vi "命令.vi"(10 "应用名称":string, 11 "选项":enum16{"归零", "自动", "退出", "关机"}(ring)) -> (3 "完成":bool)   [LabVIEW 2017]
panel:
  out "standard output 2":string caption="标准输出"
  out "匹配后偏移量 2":i32
  # "Google Chrome"
  # "SQLiteSpy.exe"
  # "Macromedia Flash Player 7.0  r14"
  # "動物連連看1.exe"
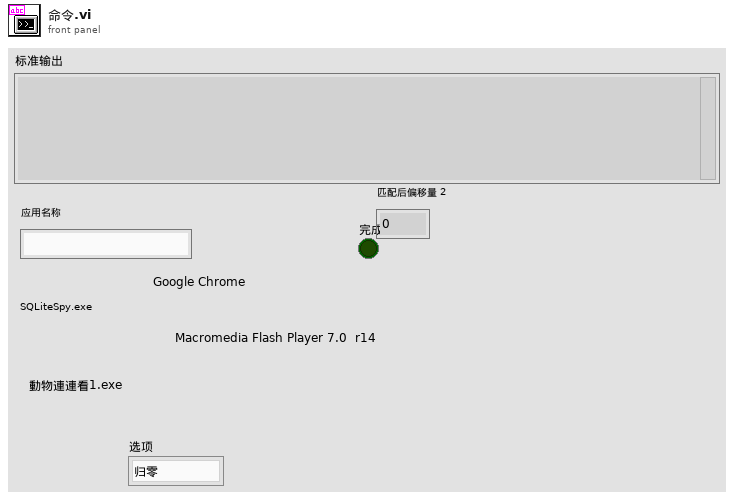
[diagram p1: front panel]
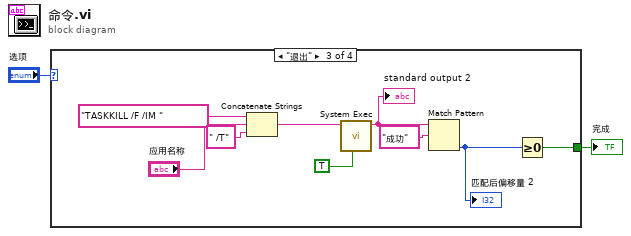
[diagram p0: block diagram]
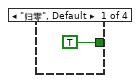
[diagram p2: hidden frame]
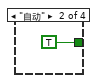
[diagram p3: hidden frame]
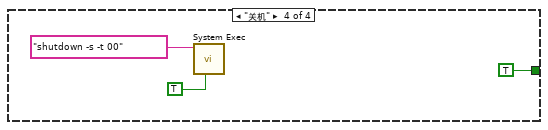
[diagram p4: hidden frame]
diagram:
  n1 = case shown="\"退出\"" "选项" {
    tunnel: [TRUE TRUE w5 TRUE] -> w2
    frame "归零", Default {
    }
    frame "自动" {
    }
    frame "退出" {
      n2 = Concatenate Strings("TASKKILL /F /IM " ("command line"), "应用名称", " /T" ("字符串")) -> (w12:string)
      n3 = call <vilib>:"System Exec.vi"("run minimized? (F)"=TRUE, "command line"=w12) -> ("standard output"=w8:string)  [unwired: 6 in, 3 out]
      "standard output 2" <- w8
      n4 = Match Pattern(string=w8, regular expression="成功" ("正则表达式")) -> (offset past match=w6:i32)  [unwired: 1 in, 3 out]
      "匹配后偏移量 2" <- w6
      n5 = Greater Or Equal To 0?(x=w6) -> (x >= 0?=w5:bool)
    }
    frame "关机" {
      n6 = call <vilib>:"System Exec.vi"("run minimized? (F)"=TRUE, "command line"="shutdown -s -t 00") -> ()  [unwired: 6 in, 4 out]
    }
  }
  "完成" <- w2
